vi "Interface.vi"(8 "error in (no error)":T1, 11 "Sim DiscreteIO in":class) -> (0 "error out":T1)   [LabVIEW 2021, in "Sim DiscreteIO.lvclass"]
uses:
  Sim DiscreteIO.lvclass
  C:/Program Files (x86)/National Instruments/LabVIEW 2021/user.lib/S2 Labs/Module Framework/Modules/Base/Module.lvclass
  Sim DiscreteIO.lvclass/Sim DiscreteIO.ctl
  <userlib>/S2 Labs/CVT Toolkit/CVT.lvclass/CVT.ctl
  Accessors/Read Initialized.vi
  13792faa-7e4f-4e90-a721-1eb543ac294b.vi
  Accessors/Read ch_labels.vi
  Accessors/Read occurrence.vi
  13792faa-7e4f-4e90-a721-1eb543ac294b.vi/1553f4ce-967c-4f57-a913-5f155bf4374d.vi
  <userlib>/S2 Labs/CVT Toolkit/Read CVT DVR.vi
  <userlib>/S2 Labs/Module Framework/Modules/Base/Get Module CVT Ref.vi
  <vilib>/Utility/error.llb/Error Cluster From Error Code.vi
  <vilib>/rvi/errors/niLvFpgaAdjustHostInterfaceError.vi
  <vilib>/rvi/interface/nirviReadWriteControl/nirviReadWriteControl.xnode
  <userlib>/S2 Labs/Module Framework/Modules/Base/Module.lvclass
  NiFpgaLv.dll
  <vilib>/rvi/interface/Simulation/niFpgaSimulationCallBeginRW.vi
panel:
  out "Stopped?":boolean
  in  "S1-DI15_F23 Pack5 Microswitch":boolean
  in  "S1-DI14_F22 Pack4 Microswitch":boolean
  in  "S1-DI13_F21 Pack3 Microswitch":boolean
  in  "S1-DI12_F20 Pack2 Microswitch":boolean
  in  "S1-DI11_F19 Pack1 Microswitch":boolean
  in  "S1-DI10_F10 DC Guard MicroSwitch":boolean
  in  "S1-DI9_F9 DC Guard MicroSwitch":boolean
  in  "S1-DI22_F30 Pack12 Microswitch":boolean
  in  "S1-DI21_F29 Pack11 Microswitch":boolean
  in  "S1-DI20_F28 Pack10 Microswitch":boolean
  in  "S1-DI19_F27 Pack9 Microswitch":boolean
  in  "S1-DI18_F26 Pack8 Microswitch":boolean
  in  "S1-DI17_F25 Pack7 Microswitch":boolean
  in  "S1-DI16_F24 Pack6 Microswitch":boolean
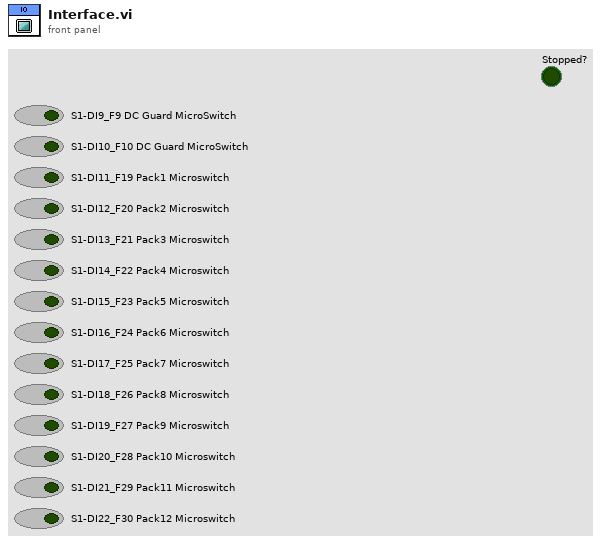
[diagram p1: front panel]
types:
  T1 = cluster{"source":string, "code":numeric, "status":boolean}
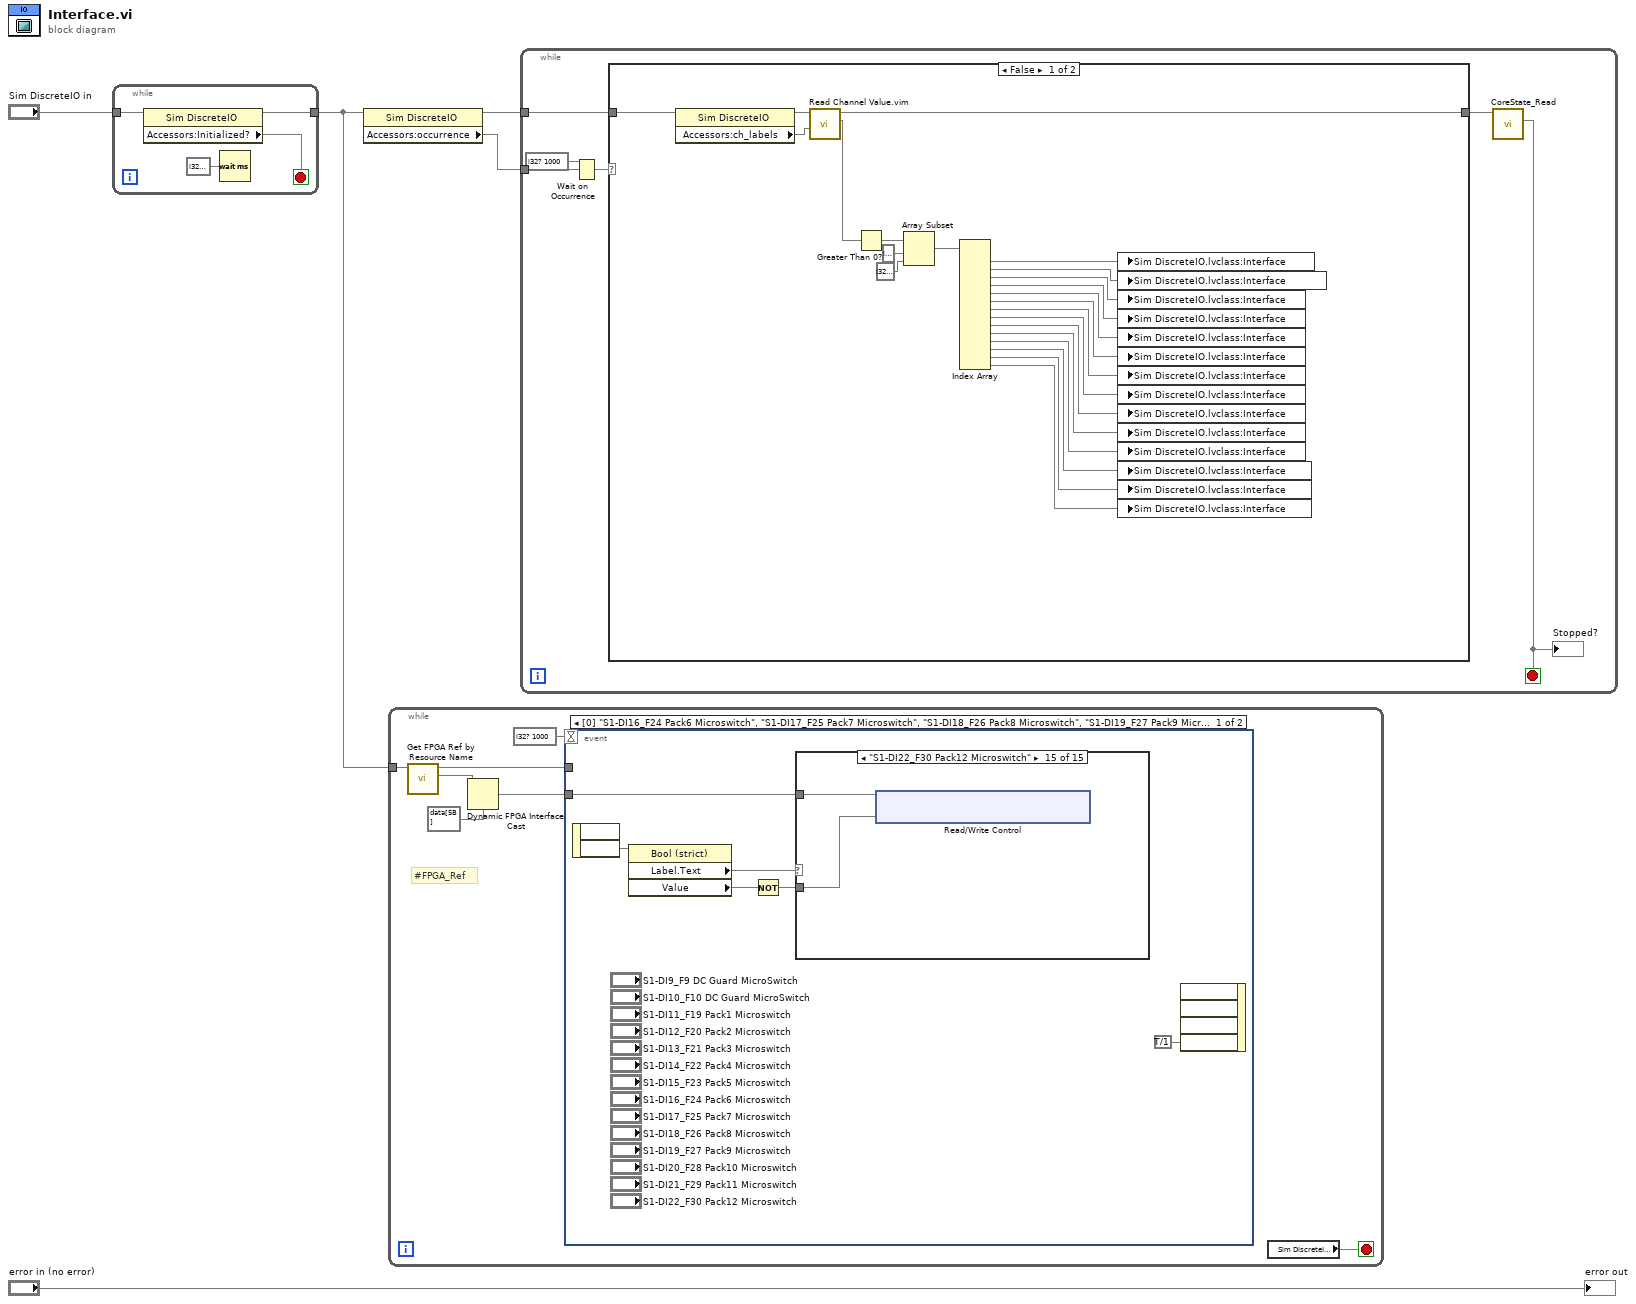
[diagram p0: block diagram]
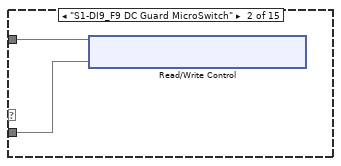
[diagram p3: hidden frame]
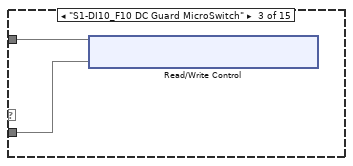
[diagram p4: hidden frame]
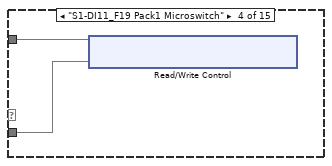
[diagram p5: hidden frame]
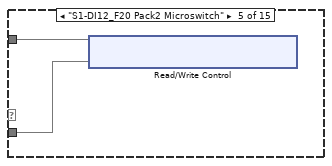
[diagram p6: hidden frame]
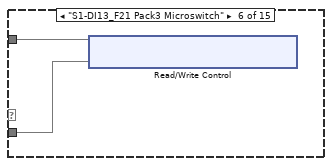
[diagram p7: hidden frame]
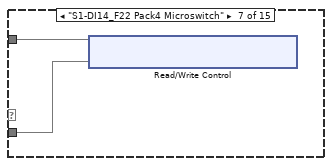
[diagram p8: hidden frame]
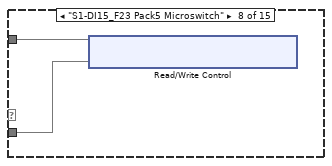
[diagram p9: hidden frame]
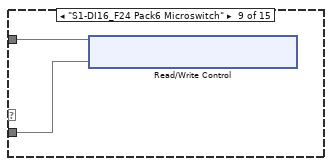
[diagram p10: hidden frame]
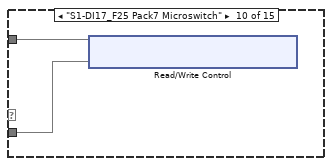
[diagram p11: hidden frame]
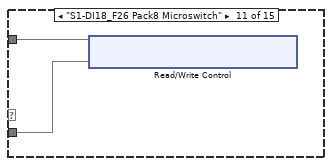
[diagram p12: hidden frame]
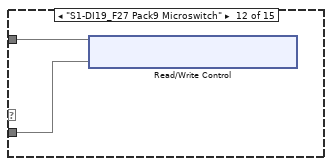
[diagram p13: hidden frame]
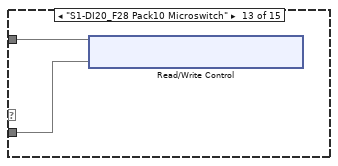
[diagram p14: hidden frame]
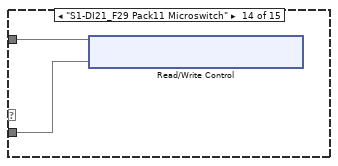
[diagram p15: hidden frame]
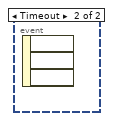
[diagram p16: hidden frame]
diagram:
  n1 = while {
    tunnel: [w9] -> w1
    tunnel: "Sim DiscreteIO in" -> [w8]
    stop <- w7 stop-if-true
    n2 = property class="Sim DiscreteIO"(reference=w8) -> (reference out=w9, "Accessors:Initialized?"=w7)  [unwired: 1 in, 1 out]
    n3 = Wait (ms)(milliseconds to wait=i32? 100) -> ()  [unwired: 1 out]
  }
  n4 = property class="Sim DiscreteIO"(reference=w1) -> (reference out=w3, "Accessors:occurrence"=w2)  [unwired: 1 in, 1 out]
  n5 = while {
    tunnel: w1 -> [w14]
    stop <- w10 stop-if-true
    # "#FPGA_Ref"
    n6 = call <userlib>:"Get FPGA Ref by Resource Name.vi"(11:w14) -> (2:w12, 3:w15)  [unwired: 7 in, 2 out]
    n7 = Dynamic FPGA Interface Cast(Session In=data[5B] ("Type"), Type=w12) -> (Session Out=w11)
    n8 = event shown="[0] \"S1-DI16_F24 Pack6 Microswitch\", \"S1-DI17_F25 Pack7 Microswitch\", \"S1-DI18_F26 Pack8 Microswitch\", \"S1-DI19_F27 Pack9 Microswitch\", \"S1-DI20_F28 Pack10 Microswitch\", \"S1-DI21_F29 Pack11 Microswitch\", \"S1-DI22_F30 Pack12 Microswitch\", \"S1-DI9_F9 DC Guard MicroSwitch\", \"S1-DI10_F10 DC Guard MicroSwitch\", \"S1-DI11_F19 Pack1 Microswitch\", \"S1-DI12_F20 Pack2 Microswitch\", \"S1-DI13_F21 Pack3 Microswitch\", \"S1-DI14_F22 Pack4 Microswitch\", \"S1-DI15_F23 Pack5 Microswitch\": Mouse Down?" {
      selector: _ -> [_ _]
      dyn-events: _ -> [_ _]
      timeout: i32? 1000 -> [_ _]
      tunnel: w15 -> [_ _]
      tunnel: w11 -> [w17 _]
      event "S1-DI16_F24 Pack6 Microswitch", "S1-DI17_F25 Pack7 Microswitch", "S1-DI18_F26 Pack8 Microswitch", "S1-DI19_F27 Pack9 Microswitch", "S1-DI20_F28 Pack10 Microswitch", "S1-DI21_F29 Pack11 Microswitch", "S1-DI22_F30 Pack12 Microswitch", "S1-DI9_F9 DC Guard MicroSwitch", "S1-DI10_F10 DC Guard MicroSwitch", "S1-DI11_F19 Pack1 Microswitch", "S1-DI12_F20 Pack2 Microswitch", "S1-DI13_F21 Pack3 Microswitch", "S1-DI14_F22 Pack4 Microswitch", "S1-DI15_F23 Pack5 Microswitch": Mouse Down? {
        n9 = event-data() -> (w21)  [unwired: 1 in, 1 out]
        n10 = property class="Bool (strict)"(reference=w21) -> ("Label.Text"=w18, "Value"=w20)  [unwired: 1 in, 2 out]
        n11 = Not(x=w20) -> (.not. x?=w19)
        n12 = case shown="\"S1-DI22_F30 Pack12 Microswitch\"" w18 {
          tunnel: w19 -> [_ w23 w25 w27 w29 w31 w33 w35 w37 w39 w41 w43 w45 w47 w49]
          tunnel: w17 -> [_ w24 w26 w28 w30 w32 w34 w36 w38 w40 w42 w44 w46 w48 w50]
          frame "False" {
          }
          frame "S1-DI9_F9 DC Guard MicroSwitch" {
            n13 = xnode "Read/Write Control"(w24, w23) -> ()  [unwired: 1 in, 2 out]
          }
          frame "S1-DI10_F10 DC Guard MicroSwitch" {
            n14 = xnode "Read/Write Control"(w26, w25) -> ()  [unwired: 1 in, 2 out]
          }
          frame "S1-DI11_F19 Pack1 Microswitch" {
            n15 = xnode "Read/Write Control"(w28, w27) -> ()  [unwired: 1 in, 2 out]
          }
          frame "S1-DI12_F20 Pack2 Microswitch" {
            n16 = xnode "Read/Write Control"(w30, w29) -> ()  [unwired: 1 in, 2 out]
          }
          frame "S1-DI13_F21 Pack3 Microswitch" {
            n17 = xnode "Read/Write Control"(w32, w31) -> ()  [unwired: 1 in, 2 out]
          }
          frame "S1-DI14_F22 Pack4 Microswitch" {
            n18 = xnode "Read/Write Control"(w34, w33) -> ()  [unwired: 1 in, 2 out]
          }
          frame "S1-DI15_F23 Pack5 Microswitch" {
            n19 = xnode "Read/Write Control"(w36, w35) -> ()  [unwired: 1 in, 2 out]
          }
          frame "S1-DI16_F24 Pack6 Microswitch" {
            n20 = xnode "Read/Write Control"(w38, w37) -> ()  [unwired: 1 in, 2 out]
          }
          frame "S1-DI17_F25 Pack7 Microswitch" {
            n21 = xnode "Read/Write Control"(w40, w39) -> ()  [unwired: 1 in, 2 out]
          }
          frame "S1-DI18_F26 Pack8 Microswitch" {
            n22 = xnode "Read/Write Control"(w42, w41) -> ()  [unwired: 1 in, 2 out]
          }
          frame "S1-DI19_F27 Pack9 Microswitch" {
            n23 = xnode "Read/Write Control"(w44, w43) -> ()  [unwired: 1 in, 2 out]
          }
          frame "S1-DI20_F28 Pack10 Microswitch" {
            n24 = xnode "Read/Write Control"(w46, w45) -> ()  [unwired: 1 in, 2 out]
          }
          frame "S1-DI21_F29 Pack11 Microswitch" {
            n25 = xnode "Read/Write Control"(w48, w47) -> ()  [unwired: 1 in, 2 out]
          }
          frame "S1-DI22_F30 Pack12 Microswitch" {
            n26 = xnode "Read/Write Control"(w50, w49) -> ()  [unwired: 1 in, 2 out]
          }
        }
        n27 = event-data(T/1 ("Discard?")) -> ()  [unwired: 4 in, 1 out]
      }
      event Timeout {
        n28 = event-data() -> ()  [unwired: 1 in, 3 out]
      }
    }
    n29 = var read "Sim DiscreteIO.lvclass:Interface.vi" item#17() -> (w10)
  }
  n30 = while {
    tunnel: w3 -> [w54]
    tunnel: w2 -> [w53]
    stop <- w56 stop-if-true
    n31 = Wait on Occurrence(2:w53, 3:i32? 1000 ("ms timeout (-1)")) -> (0:w51)  [unwired: 1 in]
    n32 = case shown="False" w51 {
      tunnel: [w79 w80] -> w55
      tunnel: w54 -> [w77 w80]
      frame 0 {
        n33 = property class="Sim DiscreteIO"(reference=w77) -> (reference out=w78, "Accessors:ch_labels"=w76)  [unwired: 1 in, 1 out]
        n34 = call "Read Channel Value.vim"(9:w76, 11:w78) -> (2:w75, 3:w79)  [unwired: 3 in, 5 out]
        n35 = Greater Than 0?(x=w75) -> (x > 0?=w73)
        n36 = Array Subset(array=w73, index=i32? 9, length=i32? 14) -> (w71)
        n37 = Index Array(array=w71) -> (element #1=w70, element #2=w69, element #3=w68, element #4=w67, element #5=w66, element #6=w65, element #7=w64, element #8=w63, element #9=w62, element #10=w61, element #11=w60, element #12=w59, element #13=w58, element #14=w57)  [unwired: 14 in]
        n38 = var write "Sim DiscreteIO.lvclass:Interface.vi" item#10(w70) -> ()
        n39 = var write "Sim DiscreteIO.lvclass:Interface.vi" item#11(w69) -> ()
        n40 = var write "Sim DiscreteIO.lvclass:Interface.vi" item#12(w68) -> ()
        n41 = var write "Sim DiscreteIO.lvclass:Interface.vi" item#13(w67) -> ()
        n42 = var write "Sim DiscreteIO.lvclass:Interface.vi" item#14(w66) -> ()
        n43 = var write "Sim DiscreteIO.lvclass:Interface.vi" item#15(w65) -> ()
        n44 = var write "Sim DiscreteIO.lvclass:Interface.vi" item#16(w64) -> ()
        n45 = var write "Sim DiscreteIO.lvclass:Interface.vi" item#3(w63) -> ()
        n46 = var write "Sim DiscreteIO.lvclass:Interface.vi" item#4(w62) -> ()
        n47 = var write "Sim DiscreteIO.lvclass:Interface.vi" item#5(w61) -> ()
        n48 = var write "Sim DiscreteIO.lvclass:Interface.vi" item#6(w60) -> ()
        n49 = var write "Sim DiscreteIO.lvclass:Interface.vi" item#7(w59) -> ()
        n50 = var write "Sim DiscreteIO.lvclass:Interface.vi" item#8(w58) -> ()
        n51 = var write "Sim DiscreteIO.lvclass:Interface.vi" item#9(w57) -> ()
      }
      frame 1 {
      }
    }
    n52 = call-dynamic "CoreState_Read.vi"(11:w55) -> (2:w56)  [unwired: 8 in, 2 out]
    "Stopped?" <- w56
  }
  "error out" <- "error in (no error)"
